vi "Calc T0 A.vi"(7 "init":bool, 8 "Pump":T1 {"P end [MPa]" format="%#_13g"; "P start [MPa]" format="%#_13g"}, 10 "U":dbl, 11 "P":dbl) -> (0 "done":bool, 2 "A":dbl, 3 "T0":dbl)   [LabVIEW 2019]
uses:
  TypeDef/Setting Pressure PI.ctl
panel:
  out "P avr":dbl
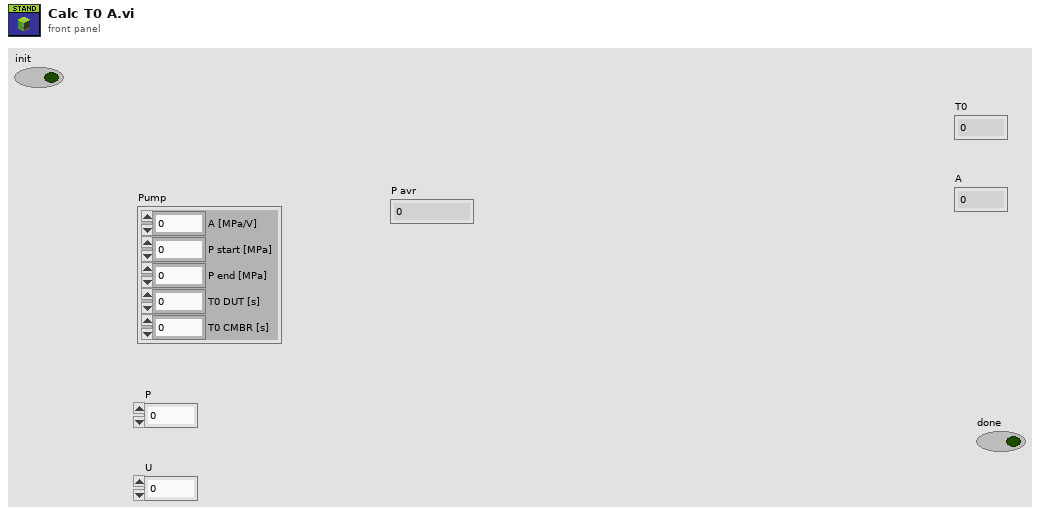
[diagram p1: front panel]
types:
  T1 = typedef "Setting Pressure PI.ctl" = cluster{"A [MPa/V]":dbl, "P start [MPa]":dbl, "P end [MPa]":dbl, "T0 DUT [s]":dbl, "T0 CMBR [s]":dbl}
  T2 = cluster{"integral P(t)":dbl, "integral U(t)":dbl, "delta P":dbl}
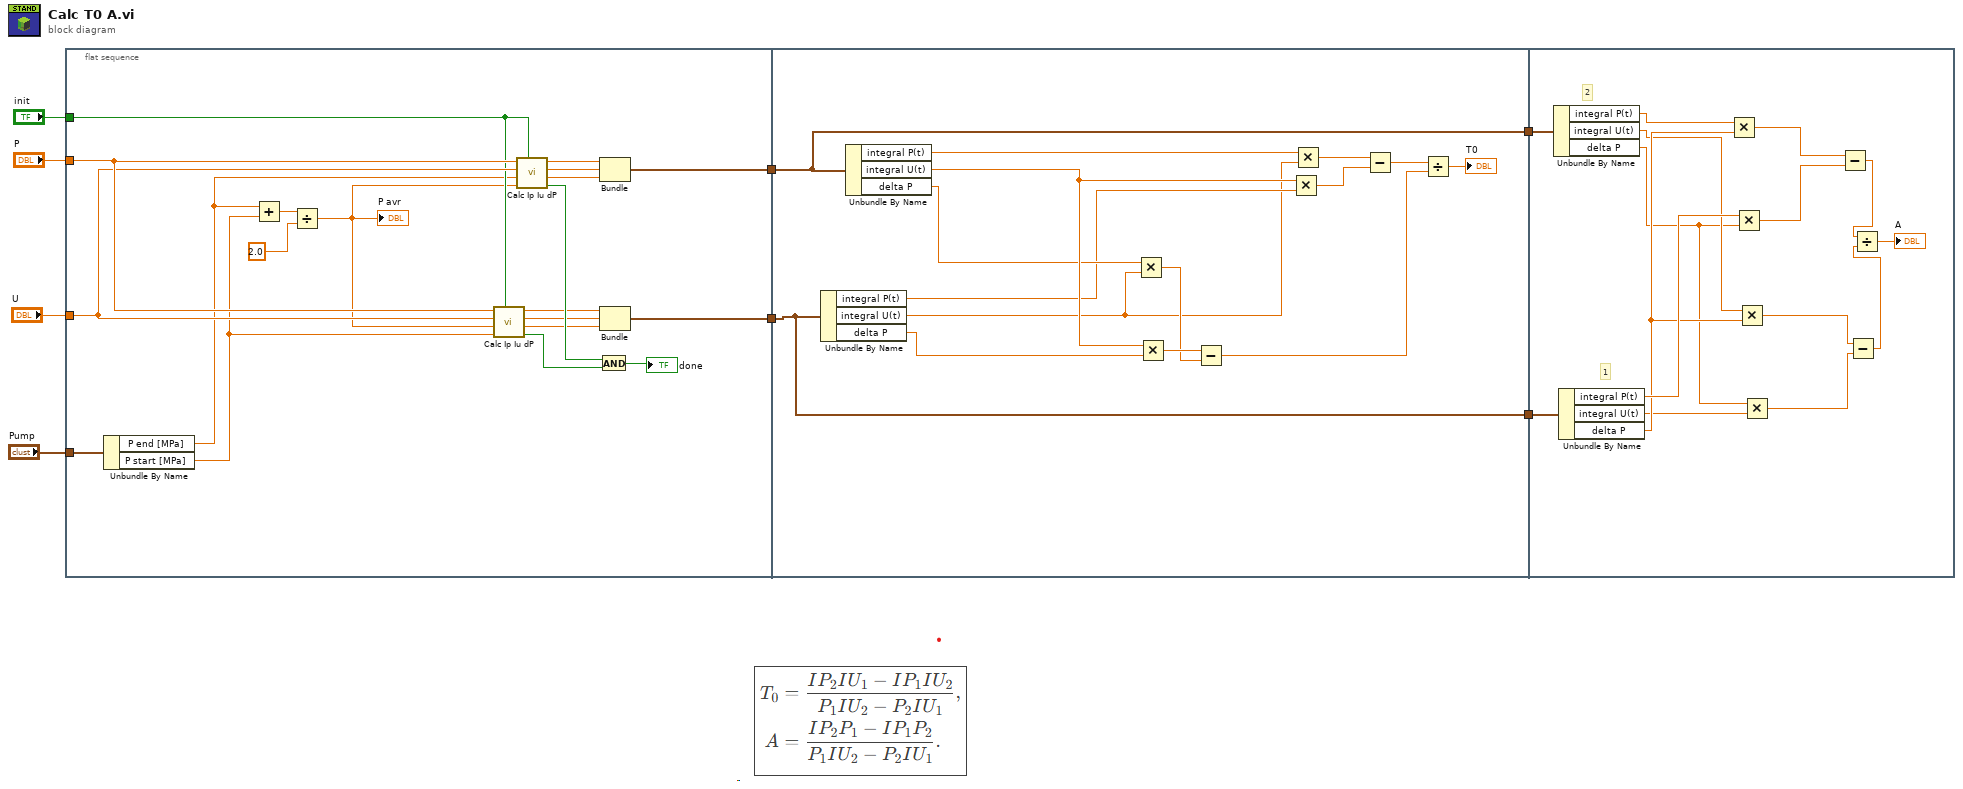
[diagram p0: block diagram]
diagram:
  n1 = flat-sequence {
    tunnel: "P" -> [w28]
    tunnel: "U" -> [w27]
    tunnel: "init" -> [w26]
    tunnel: "Pump" -> [w25]
    tunnel: [w13] -> w4
    tunnel: [w9] -> w3
    tunnel: w4 -> [w29]
    tunnel: w3 -> [w30]
    tunnel: [w30] -> w2
    tunnel: [w29] -> w1
    tunnel: w2 -> [w57]
    tunnel: w1 -> [w58]
    frame #0 {
      n2 = Unbundle By Name(w25) -> ("P end [MPa]"=w21:dbl, "P start [MPa]"=w20:dbl)
      n3 = Add(x=w21, y=w20) -> (x+y=w19:dbl)
      n4 = Divide(x=w19, y=2.0) -> (x/y=w17:dbl)
      "P avr" <- w17
      n5 = call "Calc Ip Iu dP.vi"("init"=w26, "P start [MPa]"=w20, "P end [MPa]"=w17, "U"=w27, "P"=w28) -> ("done"=w23:bool, "delta P"=w10:dbl, "integral U(t)"=w11:dbl, "integral P(t)"=w12:dbl)  [unwired: 3 in]
      n6 = call "Calc Ip Iu dP.vi"("init"=w26, "P start [MPa]"=w17, "P end [MPa]"=w21, "U"=w27, "P"=w28) -> ("done"=w24:bool, "delta P"=w14:dbl, "integral U(t)"=w15:dbl, "integral P(t)"=w16:dbl)  [unwired: 3 in]
      n7 = And(x=w24, y=w23) -> (x .and. y?=→"done":bool)
      n8 = Bundle("integral P(t)"=w16, "integral U(t)"=w15, "delta P"=w14) -> (w13:T2)  [unwired: 1 in]
      n9 = Bundle("integral P(t)"=w12, "integral U(t)"=w11, "delta P"=w10) -> (w9:T2)  [unwired: 1 in]
    }
    frame #1 {
      n10 = Unbundle By Name(w30) -> ("integral P(t)"=w33:dbl, "integral U(t)"=w32:dbl, "delta P"=w31:dbl)
      n11 = Unbundle By Name(w29) -> ("integral P(t)"=w36:dbl, "integral U(t)"=w35:dbl, "delta P"=w34:dbl)
      n12 = Multiply(x=w34, y=w32) -> (x*y=w40:dbl)
      n13 = Multiply(x=w35, y=w31) -> (x*y=w41:dbl)
      n14 = Subtract(x=w41, y=w40) -> (x-y=w38:dbl)
      n15 = Multiply(x=w35, y=w33) -> (x*y=w42:dbl)
      n16 = Multiply(x=w36, y=w32) -> (x*y=w43:dbl)
      n17 = Subtract(x=w43, y=w42) -> (x-y=w39:dbl)
      n18 = Divide(x=w39, y=w38) -> (x/y=→"T0":dbl)
    }
    frame #2 {
      # "1"
      # "2"
      n19 = Unbundle By Name(w58) -> ("integral P(t)"=w56:dbl, "integral U(t)"=w49:dbl, "delta P"=w48:dbl)
      n20 = Unbundle By Name(w57) -> ("integral P(t)"=w55:dbl, "integral U(t)"=w47:dbl, "delta P"=w50:dbl)
      n21 = Multiply(x=w56, y=w50) -> (x*y=w54:dbl)
      n22 = Multiply(x=w55, y=w48) -> (x*y=w53:dbl)
      n23 = Multiply(x=w49, y=w50) -> (x*y=w51:dbl)
      n24 = Multiply(x=w48, y=w47) -> (x*y=w52:dbl)
      n25 = Subtract(x=w54, y=w53) -> (x-y=w45:dbl)
      n26 = Subtract(x=w51, y=w52) -> (x-y=w44:dbl)
      n27 = Divide(x=w45, y=w44) -> (x/y=→"A":dbl)
    }
  }
